vi "LVProjectShortcut_Item_CanDropItem.vi"(10 "DropItem":T1, 11 "Object":T1) -> (3 "CanDrop":bool)   [LabVIEW 2017, in "LVProject Shortcut.lvlib"]
uses:
  <resource>/Framework/Providers/API/ItemRef.ctl
  LVProject Shortcut.lvlib
  <vilib>/Utility/lvfile.llb/NI_FileType.lvlib
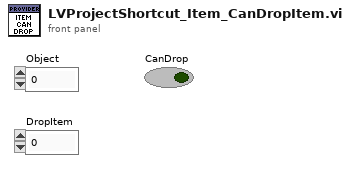
[diagram p1: front panel]
types:
  T1 = typedef "ItemRef.ctl" = u64
  T2 = typedef "mxLvNIIM.ctl" = cluster{"Item URL":string, "Item ID":string, "Item Index":i32, "Specific Type":string}
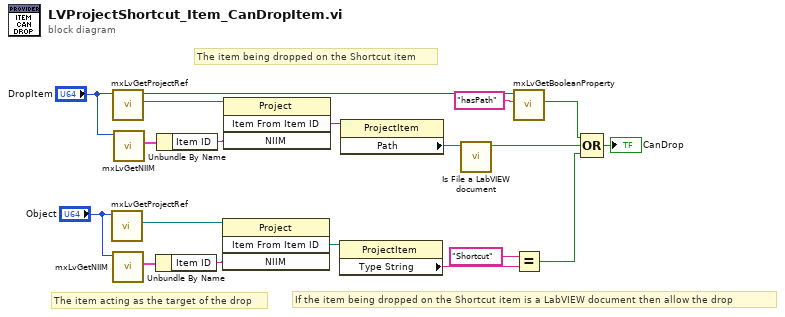
[diagram p0: block diagram]
diagram:
  # "If the item being dropped on the Shortcut item is a LabVIEW document then allow the drop"
  # "The item acting as the target of the drop"
  # "The item being dropped on the Shortcut item"
  n1 = call <resource>:"mxLvGetProjectRef.vi"("Item"="Object") -> ("Project Refnum"=w8:refnum<vi>)  [unwired: 8 in, 2 out]
  n2 = call <resource>:"mxLvGetProjectRef.vi"("Item"="DropItem") -> ("Project Refnum"=w19:refnum<vi>, "Item"=w14:T1)  [unwired: 8 in, 1 out]
  n3 = call <resource>:"mxLvGetNIIM.vi"("Item"="Object") -> ("NIIM"=w9:T2)  [unwired: 8 in, 2 out]
  n4 = call <resource>:"mxLvGetNIIM.vi"("Item"="DropItem") -> ("NIIM"=w18:T2)  [unwired: 8 in, 2 out]
  n5 = Unbundle By Name(w9) -> ("Item ID"=w10:string)
  n6 = Unbundle By Name(w18) -> ("Item ID"=w17:string)
  n7 = invoke class="Project" method="Item From Item ID"(reference=w8, "NIIM"=w10) -> ("GetItemFromNIIM"=w11:refnum<vi>)  [unwired: 2 in, 3 out]
  n8 = invoke class="Project" method="Item From Item ID"(reference=w19, "NIIM"=w17) -> ("GetItemFromNIIM"=w16:refnum<vi>)  [unwired: 2 in, 3 out]
  n9 = property class="ProjectItem"(reference=w11) -> ("Type String"=w3:string)  [unwired: 1 in, 2 out]
  n10 = property class="ProjectItem"(reference=w16) -> ("Path"=w15:path)  [unwired: 1 in, 2 out]
  n11 = call <vilib>:"Is File a LabVIEW document.vi"("path"=w15) -> ("Is LabVIEW document?"=w6:bool)  [unwired: 9 in, 1 out]
  n12 = call <resource>:"mxLvGetBooleanProperty.vi"("Tag"="hasPath", "Item"=w14) -> ("Value"=w5:bool)  [unwired: 7 in, 2 out]
  n13 = Equal?(x="Shortcut", y=w3) -> (x = y?=w1:bool)
  n14 = Compound Arithmetic op=OR(w5, w6, w1) -> (→"CanDrop":bool)
